vi "roboRIO April Tag Info AE.vi"(7 "Update":bool, 9 "Info in":dbl[](array[numeric]), 11 "name":string) -> (3 "Target Info":string)   [LabVIEW 2023]
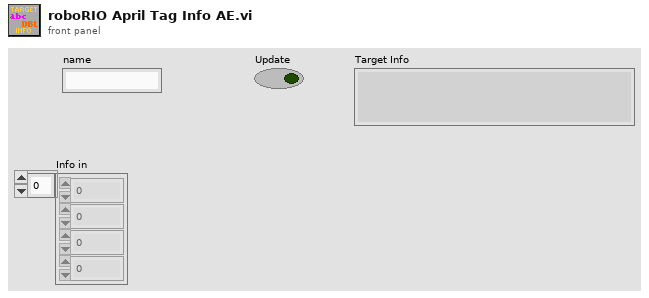
[diagram p1: front panel]
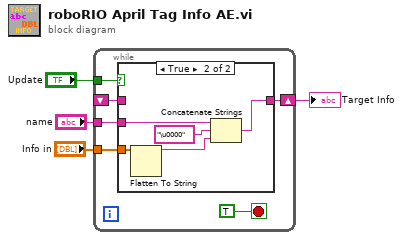
[diagram p0: block diagram]
diagram:
  n1 = while {
    tunnel: "Update" -> [w10]
    tunnel: "Info in" -> [w9]
    shift-right: [w8] -> w1
    shift-left: _ -> [w7]
    tunnel: "name" -> [w5]
    stop <- TRUE stop-if-true
    n2 = case shown="True" w10 {
      tunnel: w9 -> [_ w16]
      tunnel: [w11 w13] -> w8
      tunnel: w7 -> [w11 _]
      tunnel: w5 -> [_ w15]
      frame False {
      }
      frame True {
        n3 = Flatten To String(anything=w16) -> (data string=w14:string)  [unwired: 3 in, 2 out]
        n4 = Concatenate Strings(w15, "\u0000" ("string"), w14) -> (w13:string)
      }
    }
  }
  "Target Info" <- w1
